vi "Exit FGV.vi"(6 "Exit FGV Command":T1, 8 "Count In":i16) -> (0 "Count Out":i16)   [LabVIEW 2015]
uses:
  TypeDefs Host/Counter FGV Enum.ctl
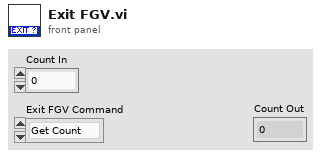
[diagram p1: front panel]
types:
  T1 = typedef "Counter FGV Enum.ctl" = enum16{"Get Count", "Set Count"}
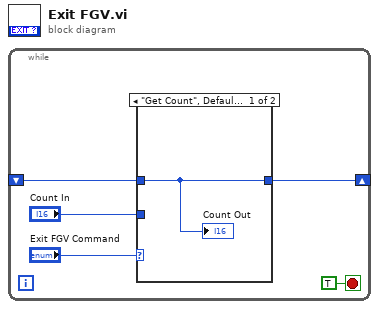
[diagram p0: block diagram]
diagram:
  n1 = while {
    shift-right: [w5] -> _
    shift-left: _ -> [w4]
    stop <- TRUE stop-if-true
    n2 = case shown="\"Get Count\", Default" "Exit FGV Command" {
      tunnel: [w6 w7] -> w5
      tunnel: w4 -> [w6 _]
      tunnel: "Count In" -> [_ w7]
      frame "Get Count", Default {
        "Count Out" <- w6
      }
      frame "Set Count" {
      }
    }
  }
